vi "Main.vi"(11 "Module Admin":refnum<class "Delacor_lib_QMH_Module Admin.lvclass">) -> ()   [LabVIEW 2022 SP3, in "Dummy.lvlib"]
doc: "This template is based off of the Queued Message Handler design pattern and the Queued Message Handler project template that ships with LabVIEW.\n\nThe main difference is that the queue is private to this module and communication between modules is performed via Broadcast and Request events.\n\nRequest events are wrapped in public API methods and are handled in the Event Handling Loop (EHL) of this VI. Any module can register for Broadcast events sent by this module. The EHL generates messages based on user interface actions.\n\nThe Message Handling Loop (MHL) processes messages generated by the EHL, or by other messages. The messages are string values, so new messages can be added easily to the Message Cases case structure in the MHL. Each message cluster can also provide an optional value for Message Data, which is a variant that can be converted to whatever message-specific data is required.\n____\nHAMPEL SOFTWARE ENGINEERING v2.6.0 (2023-12-19 10:54)"
uses:
  Dummy.lvlib
  <vilib>/Delacor/Delacor QMH/Libraries/Module Admin_class/Delacor_lib_QMH_Module Admin.lvclass
  Libraries/hse-libraries/Source/hse-dqmh/Controls/Module Display Scenarios.ctl
  Module Data--cluster.ctl
  Stop Argument--cluster.ctl
  <vilib>/Delacor/Delacor QMH/Libraries/Message Queue_class/Delacor_lib_QMH_Message Queue.lvclass/Delacor_lib_QMH_Message Queue.ctl
  <vilib>/Delacor/Delacor QMH/Libraries/Module Admin_class/Delacor_lib_QMH_Module Admin.lvclass/Delacor_lib_QMH_Module Admin.ctl
  Configure Argument--cluster.ctl
  Prepare Argument--cluster.ctl
  Request UI Display Argument--cluster.ctl
  Request UI Display (Reply Payload)--cluster.ctl
  <vilib>/Utility/miscctls.llb/LVPointTypeDef.ctl
  <vilib>/Delacor/Delacor QMH/Libraries/Message Queue_class/Delacor_lib_QMH_Enqueue Message (Single).vi
  <vilib>/Delacor/Delacor QMH/Libraries/Module Admin_class/Delacor_lib_QMH_Get External Launch.vi
  <vilib>/Utility/error.llb/Error Cluster From Error Code.vi
  <vilib>/ErrorRing/Error Ring.xnode
  <vilib>/Delacor/Delacor QMH/Libraries/Message Queue_class/Delacor_lib_QMH_Message Queue.lvclass
  Libraries/hse-libraries/Source/hse-configuration/config-ini/config-ini.lvclass
  Libraries/hse-libraries/Source/hse-dqmh/hse-dqmh.lvlib
  ExampleClone/ExampleClone.lvlib
  Framework/UI Manager/UI Manager.lvlib
panel:
  out "CLI Arguments":string[](array[string])
  in  "Btn_DisableClose":bool
  in  "Btn_EnableClose":bool
  in  "Btn_HideRTM":bool
  in  "Btn_ShowRTM":bool
  in  "Message":string
  in  "Btn Send ExampleMessage":bool
  in  "Btn Show ExampleClone BD":bool
  in  "Module Display Scenarios":T1
  in  "Btn Stop ExampleClone":bool
  in  "Btn Show ExampleClone UI":bool
  out "ExampleClone ID":i32
  in  "Btn Run ExampleClone":bool
  out "error out":errorcluster
  # "UI Demo Functions"
  # "The \"Dummy\" serves as an example of a module with HSE functionality added so it can be used inside from\nand with all the features of the HSE UI Framework.\n\nThe module features a \"Configure\" request which is automatically called from the UI Framework during\nload time. The \"Configure\" case in the MHL will then load any configuration that is needed for this module.\n\nThe module features a \"Prepare\" request which is used for preparing the module's front panel before\nshowing it. The \"Prepare\" case of the MHL is called from the \"Request UI Display\" case (which, in turn, is\ncalled by the UI Manager when loading this module into its subpanel).\n\nFurthermore, this module showcases a few of the UI Framework's features.\n\nFinally, this module facilitates the starting, stopping and  operating of an example cloneable module."
  # "Controls for operating an example cloneable module"
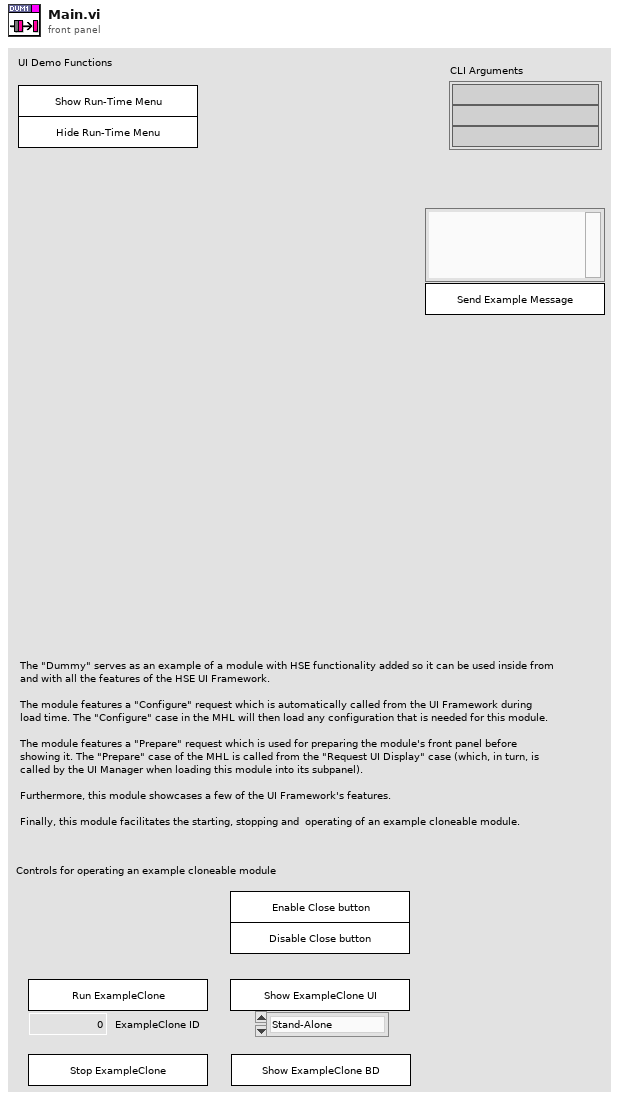
[diagram p1: front panel]
types:
  T1 = typedef "hse-dqmh.lvlib/Module Display Scenarios.ctl" = enum16{"Stand-Alone", "Managed"}
  T2 = typedef "Dummy.lvlib/Request Events--cluster.ctl" = cluster{"Stop Module":refnum<user-event>, "Show Panel":refnum<user-event>, "Hide Panel":refnum<user-event>, "Get Module Execution Status":refnum<user-event>, "Show Diagram":refnum<user-event>, "Configure":refnum<user-event>, "Prepare":refnum<user-event>, "Register for UI Login":refnum<user-event>, "Request UI Display":refnum<user-event>}
  T3 = typedef "UI Manager.lvlib/Broadcast Events--cluster.ctl" = cluster{"Module Did Init":refnum<user-event>, "Status Updated":refnum<user-event>, "Error Reported":refnum<user-event>, "Module Did Stop":refnum<user-event>, "Update Module Execution Status":refnum<user-event>, "System Message":refnum<user-event>, "Login":refnum<user-event>, "Key down":refnum<user-event>}
  T4 = typedef "Dummy.lvlib/Module Data--cluster.ctl" = cluster{"Status":string, "Clone ID's Ref":refnum<vi>}
  T5 = enum32{"invalid lock state", "Not Locked", "Locked (No Password)", "Password-protected"}
  T6 = typedef "Dummy.lvlib/Stop Argument--cluster.ctl" = cluster{"Origin":string, "Exit via Stop Module Req?":bool, "Wait for Module to stop?":bool}
  T7 = typedef "Dummy.lvlib/Configure Argument--cluster.ctl" = cluster{"Boolean":bool}
  T8 = typedef "Dummy.lvlib/Prepare Argument--cluster.ctl" = cluster{"Boolean":bool}
  T9 = typedef "Dummy.lvlib/Request UI Display Argument--cluster.ctl" = cluster{"Scenarios":T1, "Wait Notifier":refnum<notifier>, "wait for reply":bool}
  T10 = typedef "LVPointTypeDef.ctl" = cluster{"Horizontal":i16, "Vertical":i16}
  T11 = enum32{"Invalid", "Standard", "Closed", "Hidden", "Minimized", "Maximized"}
  T12 = typedef "Dummy.lvlib/Request UI Display (Reply Payload)--cluster.ctl" = cluster{"Accept?":bool, "Error":errorcluster}
  T13 = typedef "hse-dqmh.lvlib/System Message Source.ctl" = enum16{"module", "application", "network"}
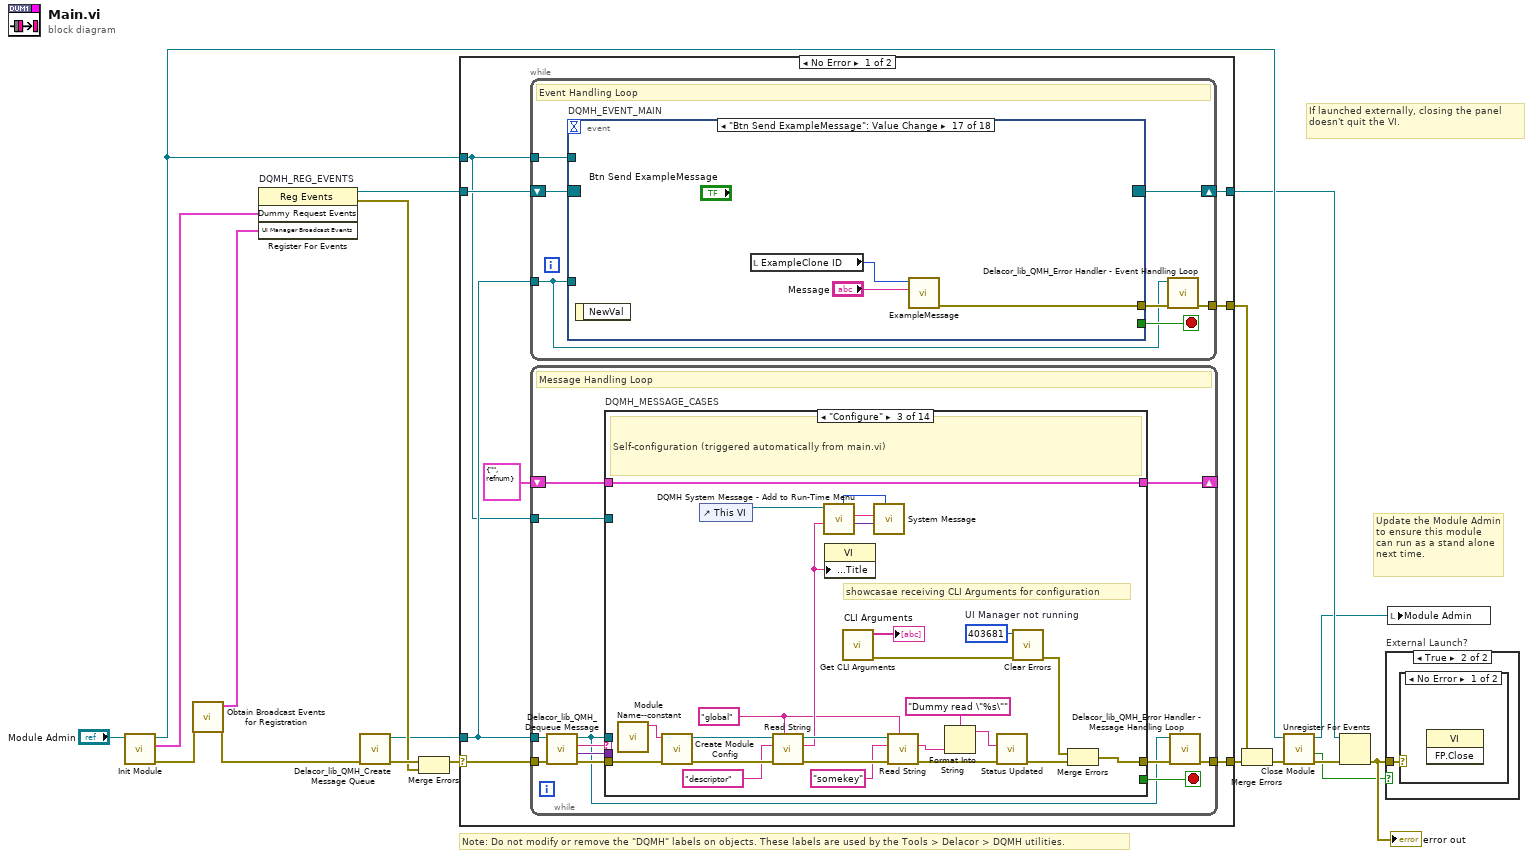
[diagram p0: block diagram]
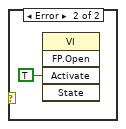
[diagram p3: hidden frame]
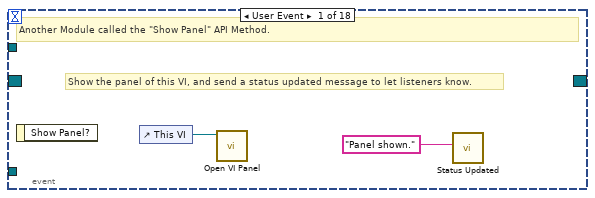
[diagram p4: hidden frame]
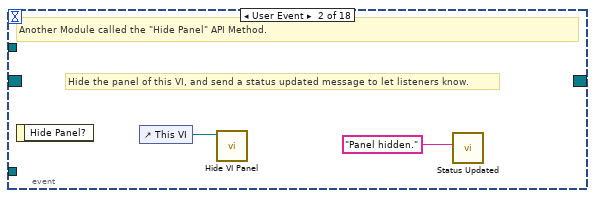
[diagram p5: hidden frame]
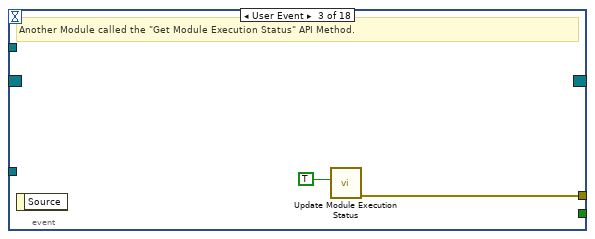
[diagram p6: hidden frame]
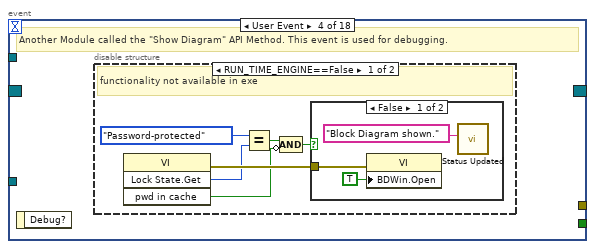
[diagram p7: hidden frame]
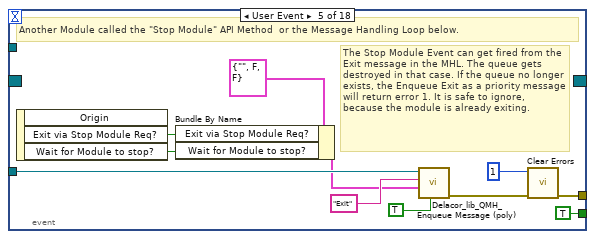
[diagram p10: hidden frame]
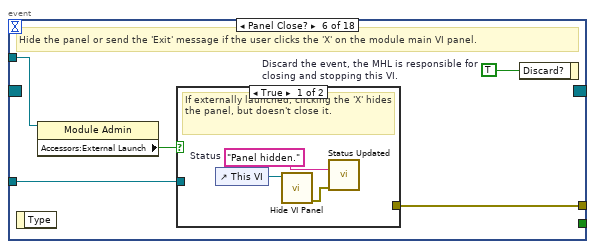
[diagram p11: hidden frame]
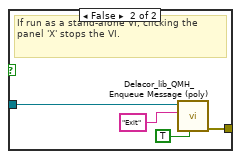
[diagram p12: hidden frame]
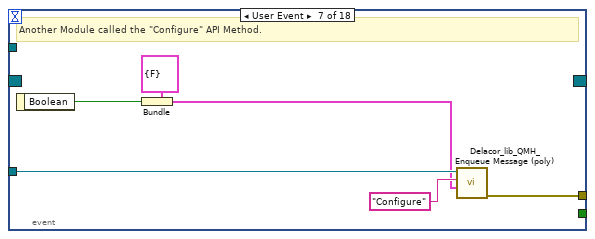
[diagram p13: hidden frame]
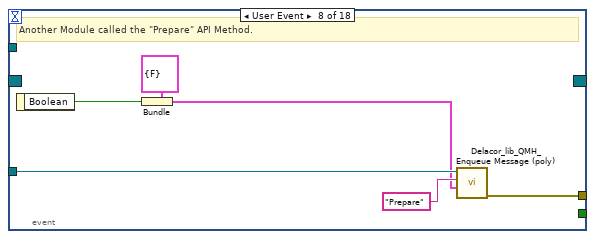
[diagram p14: hidden frame]
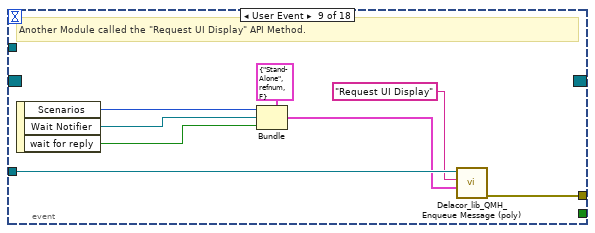
[diagram p15: hidden frame]
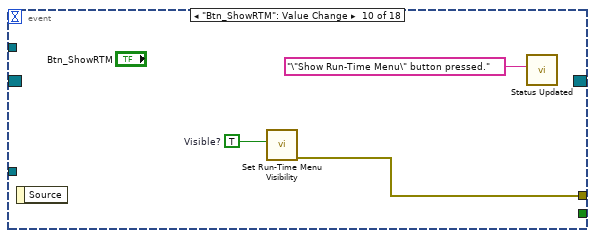
[diagram p16: hidden frame]
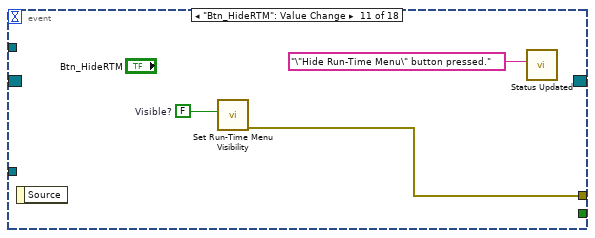
[diagram p17: hidden frame]
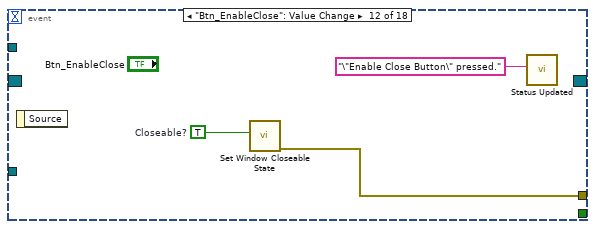
[diagram p18: hidden frame]
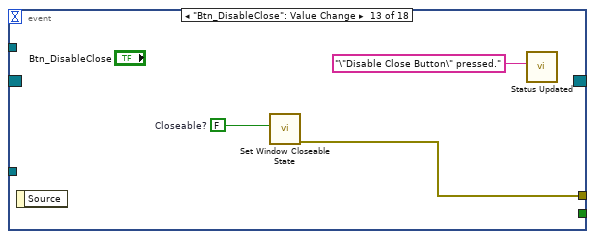
[diagram p19: hidden frame]
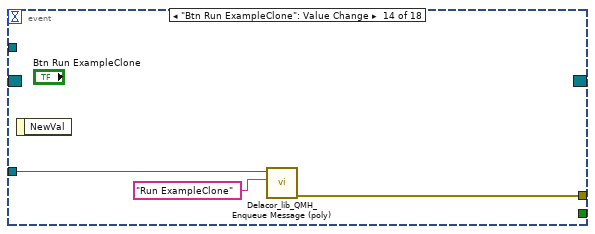
[diagram p20: hidden frame]
diagram:
  # "If launched externally, closing the panel doesn't quit the VI."
  # "Note: Do not modify or remove the \"DQMH\" labels on objects. These labels are used by the Tools > Delacor > DQMH utilities."
  # "Update the Module Admin to ensure this module can run as a stand alone next time."
  n1 = call "Init Module.vi"("Singleton Module Admin in"="Module Admin") -> ("error out"=w11:errorcluster, "Dummy Request Events"=w6:T2, "Singleton Module Admin out"=w9:refnum<class "Delacor_lib_QMH_Module Admin.lvclass">)  [unwired: 8 in]
  n2 = call "Obtain Broadcast Events for Registration.vi"("error in (no error)"=w11) -> ("error out"=w10:errorcluster, "UI Manager Broadcast Events"=w1:T3)  [unwired: 8 in, 1 out]
  n3 = register-events "DQMH_REG_EVENTS"(w6, w1) -> (reference out=w7:refnum<event-registration>, error out=w12:errorcluster)  [unwired: 2 in]
  n4 = call <vilib>:"Delacor_lib_QMH_Create Message Queue.vi"("error in"=w10) -> ("error out"=w14:errorcluster, "Message Queue"=w5:refnum<class "Delacor_lib_QMH_Message Queue.lvclass">)  [unwired: 9 in]
  n5 = Merge Errors(w14, w12) -> (w13:errorcluster)
  n6 = case shown="No Error" w13 {
    selector: w13 -> [w25 w297]
    tunnel: [w27 w297] -> w19
    tunnel: [w24 w294] -> w8
    tunnel: w7 -> [w22 w294]
    tunnel: w5 -> [w21 w289]
    tunnel: [w26 _] -> w17
    tunnel: w9 -> [w20 w290]
    frame No Error {
      n7 = while {
        tunnel: w21 -> [w28]
        shift-right: [w31] -> w24
        shift-left: w22 -> [w32]
        tunnel: [w33] -> w26
        tunnel: w20 -> [w29]
        stop <- w30 stop-if-true
        # "Event Handling Loop"
        n8 = event "DQMH_EVENT_MAIN" shown="[16] \"Btn Send ExampleMessage\": Value Change" {
          selector: w32 -> [_ _ _ _ _ _ _ _ _ _ _ _ _ _ _ _ _ _]
          dyn-events: [_ _ _ _ _ _ _ _ _ _ _ _ _ _ _ _ _ _] -> w31
          timeout: _ -> [_ _ _ _ _ _ _ _ _ _ _ _ _ _ _ _ _ _]
          tunnel: [_ _ _ _ TRUE ("Discard?") _ _ _ _ _ _ _ _ _ _ _ _ _] -> w30
          tunnel: w28 -> [_ _ _ _ w56 w63 w77 w83 w91 _ _ _ _ w105 w108 w112 _ w118]
          tunnel: [_ _ w40 _ w59 w65 w78 w84 w92 w95 w98 w101 w104 w107 w110 w114 w117 w120] -> w34
          tunnel: w29 -> [_ _ _ _ _ w62 _ _ _ _ _ _ _ _ _ _ _ _]
          event User Event {
            # "Show the panel of this VI, and send a status updated message to let listeners know."
            # "Another Module called the \"Show Panel\" API Method."
            n9 = event-data() -> ()  [unwired: 1 in, 1 out]
            n10 = control-ref of="This VI"() -> (w36:refnum<vi>)
            n11 = call "Open VI Panel.vi"("VI"=w36) -> ()  [unwired: 10 in, 1 out]
            n12 = call "Status Updated.vi"("Status"="Panel shown." ("format string")) -> ()  [unwired: 10 in, 1 out]
          }
          event User Event {
            # "Hide the panel of this VI, and send a status updated message to let listeners know."
            # "Another Module called the \"Hide Panel\" API Method."
            n13 = event-data() -> ()  [unwired: 1 in, 1 out]
            n14 = control-ref of="This VI"() -> (w38:refnum<vi>)
            n15 = call "Hide VI Panel.vi"("VI"=w38) -> ()  [unwired: 10 in, 1 out]
            n16 = call "Status Updated.vi"("Status"="Panel hidden." ("format string")) -> ()  [unwired: 10 in, 1 out]
          }
          event User Event {
            # "Another Module called the \"Get Module Execution Status\" API Method."
            n17 = event-data() -> ()  [unwired: 1 in, 1 out]
            n18 = call "Update Module Execution Status.vi"("Running?"=TRUE) -> ("error out"=w40:errorcluster)  [unwired: 10 in]
          }
          event User Event {
            # "Another Module called the \"Show Diagram\" API Method. This event is used for debugging."
            n19 = event-data() -> ()  [unwired: 1 in, 1 out]
            n20 = disable-structure shown="RUN_TIME_ENGINE==False" {
              frame condition #0 (active) {
                # "functionality not available in exe"
                n21 = invoke on="Invoke Node" class="VI" method="Lock State.Get"() -> (error out=w46:errorcluster, "Get Lock State"=w45:T5, "pwd in cache"=w42:bool)  [unwired: 4 in, 1 out]
                n22 = Equal?(x=T5."Password-protected", y=w45) -> (x = y?=w43:bool)
                n23 = Compound Arithmetic op=AND(w43, invert w42) -> (w41:bool)
                n24 = case shown="False" w41 {
                  tunnel: w46 -> [w49 _]
                  frame False {
                    n25 = property on="Property Node" class="VI"(error in=w49, "BDWin.Open"=TRUE ("Block Diagram Window:Open")) -> ()  [unwired: 1 in, 2 out]
                    n26 = call "Status Updated.vi"("Status"="Block Diagram shown." ("format string")) -> ()  [unwired: 10 in, 1 out]
                  }
                  frame True {
                    # "Password-protected VI, and the password is not in the cache. Do not show the diagram."
                  }
                }
              }
              frame condition #1 {
              }
            }
          }
          event User Event {
            # "The Stop Module Event can get fired from the Exit message in the MHL. The queue gets destroyed in that case. If the queue no longer exists, the Enqueue Exit as a priority message will return error 1. It is safe to ignore, because the module is already exiting."
            # "Another Module called the \"Stop Module\" API Method  or the Message Handling Loop below."
            n27 = event-data() -> ("Exit via Stop Module Req?"=w52:bool, "Wait for Module to stop?"=w51:bool)  [unwired: 1 in, 1 out]
            n28 = Bundle By Name(cluster=T6 {"Origin"="", "Exit via Stop Module Req?"=FALSE, "Wait for Module to stop?"=FALSE} ("Stop Argument"), "Exit via Stop Module Req?"=w52, "Wait for Module to stop?"=w51) -> (w50:T6)
            n29 = call-poly <vilib>:"Delacor_lib_QMH_Enqueue Message (poly).vi"("Priority Message? (F)"=TRUE, "Message Data"=w50, "Message"="Exit", "Message Queue in"=w56) -> ("error out"=w60:errorcluster)  [unwired: 6 in, 1 out]
            n30 = call <vilib>:"Clear Errors.vi"("error in (no error)"=w60, "specific error code to clear (0: all)"=1) -> ("error out"=w59:errorcluster)  [unwired: 4 in, 1 out]
          }
          event Panel Close? {
            w64 = TRUE  # Discard the event, the MHL is responsible for closing and stopping this VI.
            # "Hide the panel or send the 'Exit' message if the user clicks the 'X' on the module main VI panel."
            n31 = event-data() -> ()  [unwired: 1 in, 1 out]
            n32 = property on="Property Node" class="Module Admin"(reference=w62) -> ("Accessors:External Launch"=w61:bool)  [unwired: 1 in, 2 out]
            n33 = case shown="True" w61 {
              tunnel: w63 -> [_ w71]
              tunnel: [_ w72] -> w65
              frame True {
                w67 = "Panel hidden."  # Status
                # "If externally launched, clicking the 'X' hides the panel, but doesn't close it."
                n34 = control-ref of="This VI"() -> (w68:refnum<vi>)
                n35 = call "Hide VI Panel.vi"("VI"=w68) -> ("error out"=w66:errorcluster)  [unwired: 10 in]
                n36 = call "Status Updated.vi"("error in (no error)"=w66, "Status"=w67) -> ()  [unwired: 9 in, 1 out]
              }
              frame False {
                # "If run as a stand-alone VI, clicking the panel 'X' stops the VI."
                n37 = call-poly <vilib>:"Delacor_lib_QMH_Enqueue Message (poly).vi"("Priority Message? (F)"=TRUE, "Message"="Exit", "Message Queue in"=w71) -> ("error out"=w72:errorcluster)  [unwired: 7 in, 1 out]
              }
            }
            n38 = event-data ("Event Filter Node")("Discard?"=w64) -> ()  [unwired: 1 in, 1 out]
          }
          event User Event {
            # "Another Module called the \"Configure\" API Method."
            n39 = event-data() -> ("Boolean"=w73:bool)  [unwired: 1 in]
            n40 = Bundle(cluster=T7 {"Boolean"=FALSE} ("Configure Argument"), "Boolean"=w73) -> (w74:T7)
            n41 = call-poly <vilib>:"Delacor_lib_QMH_Enqueue Message (poly).vi"("Message Data"=w74, "Message"="Configure", "Message Queue in"=w77) -> ("error out"=w78:errorcluster)  [unwired: 7 in, 1 out]
          }
          event User Event {
            # "Another Module called the \"Prepare\" API Method."
            n42 = event-data() -> ("Boolean"=w79:bool)  [unwired: 1 in]
            n43 = Bundle(cluster=T8 {"Boolean"=FALSE} ("Prepare Argument"), "Boolean"=w79) -> (w80:T8)
            n44 = call-poly <vilib>:"Delacor_lib_QMH_Enqueue Message (poly).vi"("Message Data"=w80, "Message"="Prepare", "Message Queue in"=w83) -> ("error out"=w84:errorcluster)  [unwired: 7 in, 1 out]
          }
          event User Event {
            # "Another Module called the \"Request UI Display\" API Method."
            n45 = event-data() -> ("Scenarios"=w87:T1, "Wait Notifier"=w86:refnum<notifier>, "wait for reply"=w85:bool)  [unwired: 1 in]
            n46 = Bundle(cluster=T9 {"Scenarios"=enum."Stand-Alone", "Wait Notifier"=refnum, "wait for reply"=FALSE} ("Display Module UI Argument"), "Scenarios"=w87, "Wait Notifier"=w86, "wait for reply"=w85) -> (w88:T9)
            n47 = call-poly <vilib>:"Delacor_lib_QMH_Enqueue Message (poly).vi"("Message Data"=w88, "Message"="Request UI Display", "Message Queue in"=w91) -> ("error out"=w92:errorcluster)  [unwired: 7 in, 1 out]
          }
          event "Btn_ShowRTM": Value Change {
            w94 = TRUE  # Visible?
            n48 = event-data() -> ()  [unwired: 1 in, 1 out]
            n49 = call "Set Run-Time Menu Visibility.vi"("Visible?"=w94) -> ("error out"=w95:errorcluster)  [unwired: 10 in]
            n50 = call "Status Updated.vi"("Status"="\"Show Run-Time Menu\" button pressed.") -> ()  [unwired: 10 in, 1 out]
          }
          event "Btn_HideRTM": Value Change {
            w97 = FALSE  # Visible?
            n51 = event-data() -> ()  [unwired: 1 in, 1 out]
            n52 = call "Set Run-Time Menu Visibility.vi"("Visible?"=w97) -> ("error out"=w98:errorcluster)  [unwired: 10 in]
            n53 = call "Status Updated.vi"("Status"="\"Hide Run-Time Menu\" button pressed.") -> ()  [unwired: 10 in, 1 out]
          }
          event "Btn_EnableClose": Value Change {
            w100 = TRUE  # Closeable?
            n54 = event-data() -> ()  [unwired: 1 in, 1 out]
            n55 = call "Set Window Closeable State.vi"("Closeable?"=w100) -> ("error out"=w101:errorcluster)  [unwired: 10 in]
            n56 = call "Status Updated.vi"("Status"="\"Enable Close Button\" pressed.") -> ()  [unwired: 10 in, 1 out]
          }
          event "Btn_DisableClose": Value Change {
            w103 = FALSE  # Closeable?
            n57 = event-data() -> ()  [unwired: 1 in, 1 out]
            n58 = call "Set Window Closeable State.vi"("Closeable?"=w103) -> ("error out"=w104:errorcluster)  [unwired: 10 in]
            n59 = call "Status Updated.vi"("Status"="\"Disable Close Button\" pressed.") -> ()  [unwired: 10 in, 1 out]
          }
          event "Btn Run ExampleClone": Value Change {
            n60 = event-data() -> ()  [unwired: 1 in, 1 out]
            n61 = call-poly <vilib>:"Delacor_lib_QMH_Enqueue Message (poly).vi"("Message"="Run ExampleClone", "Message Queue in"=w105) -> ("error out"=w107:errorcluster)  [unwired: 8 in, 1 out]
          }
          event "Btn Show ExampleClone BD": Value Change {
            n62 = event-data() -> ()  [unwired: 1 in, 1 out]
            n63 = call-poly <vilib>:"Delacor_lib_QMH_Enqueue Message (poly).vi"("Message"="Show ExampleClone BD", "Message Queue in"=w108) -> ("error out"=w110:errorcluster)  [unwired: 8 in, 1 out]
          }
          event "Btn Show ExampleClone UI": Value Change {
            n64 = event-data() -> ()  [unwired: 1 in, 1 out]
            n65 = call-poly <vilib>:"Delacor_lib_QMH_Enqueue Message (poly).vi"("Message Data"="Module Display Scenarios", "Message"="Display ExampleClone UI", "Message Queue in"=w112) -> ("error out"=w114:errorcluster)  [unwired: 7 in, 1 out]
          }
          event "Btn Send ExampleMessage": Value Change {
            n66 = event-data() -> ()  [unwired: 1 in, 1 out]
            n67 = local read "ExampleClone ID"() -> (w115:i32)
            n68 = call "ExampleMessage.vi"("ExampleMessage"="Message", "Module ID"=w115) -> ("error out"=w117:errorcluster)  [unwired: 9 in]
          }
          event "Btn Stop ExampleClone": Value Change {
            n69 = event-data() -> ()  [unwired: 1 in, 1 out]
            n70 = call-poly <vilib>:"Delacor_lib_QMH_Enqueue Message (poly).vi"("Message"="Stop ExampleClone", "Message Queue in"=w118) -> ("error out"=w120:errorcluster)  [unwired: 8 in, 1 out]
          }
        }
        n71 = call-dynamic "Delacor_lib_QMH_Error Handler - Event Handling Loop.vi"("error in"=w34, "Message Queue in"=w28) -> ("dup error in"=w33:errorcluster)  [unwired: 8 in, 1 out]
      }
      n72 = while {
        tunnel: w21 -> [w123]
        shift-right: [w127] -> _
        shift-left: T4 {"Status"="", "Clone ID's Ref"=refnum} ("Data Cluster") -> [w128]
        tunnel: w25 -> [w131]
        tunnel: [w129] -> w27
        tunnel: w20 -> [w121]
        stop <- w126 stop-if-true
        # "Message Handling Loop"
        n73 = call-dynamic "Delacor_lib_QMH_Dequeue Message.vi"("error in"=w131, "Message Queue in"=w123) -> ("error out"=w130:errorcluster, "Message Data"=w124:variant, "Message"=w125:string, "Message Queue out"=w122:refnum<class "Delacor_lib_QMH_Message Queue.lvclass">)  [unwired: 6 in]
        n74 = case "DQMH_MESSAGE_CASES" shown="\"Configure\"" w125 {
          selector: w125 -> [_ _ _ _ _ _ _ _ _ _ _ _ _ w276]
          tunnel: w122 -> [_ _ _ _ _ _ _ _ _ _ _ w244 w267 _]
          tunnel: w130 -> [w149 w153 w159 w180 w191 w206 w214 w220 w229 w237 w241 w251 w274 w278]
          tunnel: [w148 w153 w163 w180 w189 w205 w216 w222 w231 w238 w241 w247 w271 w279] -> w132
          tunnel: w128 -> [w134 w152 w175 w179 w188 w204 w211 w219 w227 w235 w240 w246 w266 w277]
          tunnel: [w134 w152 w175 w179 w188 w204 w211 w219 w227 w235 w240 w246 w266 w277] -> w127
          tunnel: [_ _ _ _ _ _ _ _ _ _ _ _ w265 _] -> w126
          tunnel: w124 -> [_ _ _ _ w187 _ _ _ w226 _ _ w245 w264 _]
          tunnel: w121 -> [w139 _ _ _ _ _ _ _ _ _ _ w243 w259 _]
          frame "Initialize" {
            # "Initialize - Any operation that needs to be done before the module can receive messages. Synchronize Caller Events.vi will inform Start Module.vi that the module has launched and is ready to receive messages. Module Did Init.vi will broadcast that the module initialized."
            n75 = call "Synchronize Caller Events.vi"("error in (no error)"=w149, "Singleton Module Admin in"=w139) -> ("error out"=w147:errorcluster, "Singleton Module Admin out"=w136:refnum<class "Delacor_lib_QMH_Module Admin.lvclass">)  [unwired: 8 in]
            n76 = property on="Property Node" class="Module Admin"(reference=w136) -> ("Accessors:External Launch"=w143:bool)  [unwired: 1 in, 2 out]
            n77 = Select(t=T11."Hidden" ("State"), s=w143, f=T11."Standard" ("State")) -> (s? t:f=w140:T11)
            n78 = call "Module Name--constant.vi"() -> ("Module Name"=w146:string)  [unwired: 11 in]
            n79 = property on="Property Node" class="VI"("Front Panel.Title"=w146) -> (reference out=w145:refnum<vi>, error out=w151:errorcluster)  [unwired: 2 in]
            n80 = call "Module Name--constant.vi"() -> ("Module Name"=w137:string)  [unwired: 11 in]
            n81 = local write "ExampleClone ID"(-1 ("ExampleClone ID")) -> ()
            n82 = invoke on="Invoke Node" class="VI" method="FP.Open"(reference=w145, error in=w151, "State"=w140) -> (reference out=w144:refnum<vi>, error out=w150:errorcluster)  [unwired: 2 in, 3 out]
            n83 = call "Module Did Init.vi"("error in (no error)"=w147, "Initialized?"=TRUE, "Origin"=w137) -> ("error out"=w148:errorcluster)  [unwired: 8 in]
            n84 = invoke on="Invoke Node" class="VI" method="FP.Center"(reference=w144, error in=w150) -> ()  [unwired: 1 in, 3 out]
            n85 = property on="Pane" class="Pane"("Origin"=T10 {"Horizontal"=0, "Vertical"=0}) -> ()  [unwired: 2 in, 2 out]
          }
          frame "--- Module Specific ---" {
            # "Separator -- The following cases handle messages specific to this Module."
          }
          frame "Configure" {
            w160 = 403681  # UI Manager not running
            w155 = "global" ("Section")
            # "showcasae receiving CLI Arguments for configuration"
            # "Self-configuration (triggered automatically from main.vi)"
            n86 = call "Module Name--constant.vi"() -> ("Module Name"=w157:string)  [unwired: 11 in]
            n87 = call "Create Module Config.vi"("error in"=w159, "DQMH Module Name"=w157) -> ("error out"=w158:errorcluster, "config-ini out"=w156:refnum<class "config-ini.lvclass">)  [unwired: 8 in]
            n88 = control-ref of="This VI"() -> (w165:refnum<vi>)
            n89 = call-dynamic "Read String.vi"("Section"=w155, "error in"=w158, "Key"="descriptor", "config-base in"=w156) -> ("error out"=w176:errorcluster, "Value"=w166:string, "config-base out"=w167:refnum<class "config-ini.lvclass">)  [unwired: 5 in]
            n90 = call "DQMH System Message - Add to Run-Time Menu.vi"("Module Descriptor"=w166, "Main VI Reference"=w165) -> ("Payload"=w169:variant, "Identifier"=w168:string, "Source"=w170:T13)  [unwired: 7 in]
            n91 = property on="Property Node" class="VI"("Front Panel.Title"=w166) -> ()  [unwired: 2 in, 2 out]
            n92 = call "Get CLI Arguments.vi"() -> ("error out"=w162:errorcluster, "CLI Arguments"=→"CLI Arguments":string[])  [unwired: 9 in, 1 out]
            n93 = call "System Message.vi"("S. Message Source"=w170, "Payload"=w169, "Identifier"=w168) -> ()  [unwired: 8 in, 1 out]
            n94 = call-dynamic "Read String.vi"("Section"=w155, "error in"=w176, "Key"="somekey", "config-base in"=w167) -> ("error out"=w178:errorcluster, "Value"=w171:string)  [unwired: 5 in, 1 out]
            n95 = Format Into String(format string="Dummy read \"%s\"", w171) -> (resulting string=w172:string)  [unwired: 2 in, 1 out]
            n96 = call "Status Updated.vi"("error in (no error)"=w178, "Status"=w172) -> ("error out"=w177:errorcluster)  [unwired: 9 in]
            n97 = call <vilib>:"Clear Errors.vi"("error in (no error)"=w162, "specific error code to clear (0: all)"=w160) -> ("error out"=w161:errorcluster)  [unwired: 4 in, 1 out]
            n98 = Merge Errors(w161, w177) -> (w163:errorcluster)
          }
          frame "Prepare" {
            # "Prepare (the UI of the) module for display"
          }
          frame "Request UI Display" {
            # "Requests the module to display its UI as specified in <b>Scenario</b>:\n\"managed\" => in the UI Manager's subpanel\n\"stand-alone\" => as a separate window"
            n99 = Variant To Data(error in=w191, type=T9 {"Scenarios"=enum."Stand-Alone", "Wait Notifier"=refnum, "wait for reply"=FALSE} ("Request UI Display Argument"), Variant=w187) -> (data=w185:T9, error out=w190:errorcluster)
            n100 = Unbundle By Name(w185) -> ("Scenarios"=w181:T1, "Wait Notifier"=w184:refnum<notifier>, "wait for reply"=w183:bool)
            n101 = control-ref of="This VI"() -> (w182:refnum<vi>)
            n102 = case shown="\"Managed\"" w181 {
              tunnel: w182 -> [w193 w195]
              tunnel: [w194 w199] -> w192
              frame "Stand-Alone", Default {
                n103 = call "Open VI Panel.vi"("VI"=w193) -> ("error out"=w194:errorcluster)  [unwired: 10 in]
              }
              frame "Managed" {
                n104 = call "DQMH System Message - Ready for Display.vi"("Main VI Reference"=w195) -> ("Payload"=w198:variant, "Identifier"=w197:string, "Source"=w196:T13)  [unwired: 8 in]
                n105 = call "System Message.vi"("S. Message Source"=w196, "Payload"=w198, "Identifier"=w197) -> ("error out"=w199:errorcluster)  [unwired: 8 in]
              }
            }
            n106 = case shown="True" w183 {
              tunnel: w184 -> [_ w202]
              tunnel: w192 -> [_ w203]
              frame False {
              }
              frame True {
                n107 = Bundle By Name(cluster=T12 {"Accept?"=FALSE, "Error"={"status"=FALSE, "code"=0, "source"=""}} ("Request UI Display (Reply Payload)"), "Error"=w203) -> (w200:T12)
                n108 = Send Notification(notification=w200, notifier=w202) -> ()  [unwired: 1 in, 2 out]
              }
            }
            n109 = Merge Errors(w190, w192) -> (w189:errorcluster)
          }
          frame "---ExampleClone Functions---" {
            # "ExampleClone is a showcase for how the HSE DQMH functions work with cloneable modules"
            n110 = Merge Errors(w206) -> (w205:errorcluster)
          }
          frame "Run ExampleClone" {
            # "3. configure"
            # "2. register with framework"
            # "1. start module"
            # "ExampleClone is a showcase for how the HSE DQMH functions work with cloneable modules.\nBeware: It's important to register the clone with the Framework!"
            n111 = call "Start Module.vi"("error in (no error)"=w214) -> ("error out"=w215:errorcluster, "Wait for Event Sync?"=w210:bool, "Module ID"=w209:i32)  [unwired: 7 in, 1 out]
            n112 = call "Synchronize Module Events.vi"("error in (no error)"=w215, "Wait for Event Sync?"=w210, "Module ID"=w209) -> ("error out"=w217:errorcluster, "Module ID (dup)"=w208:i32)  [unwired: 7 in]
            "ExampleClone ID" <- w208
            n113 = control-ref of="This Application"() -> (w207:refnum<vi>)
            n114 = call "Register Clone with Framework.vi"("error in (no error)"=w217, "Application in"=w207) -> ("error out"=w213:errorcluster)  [unwired: 9 in]
            n115 = call "Configure.vi"("error in (no error)"=w213, "Module ID"=w208) -> ("error out"=w212:errorcluster)  [unwired: 9 in]
            n116 = Merge Errors(w212) -> (w216:errorcluster)
          }
          frame "Show ExampleClone BD" {
            # "ExampleClone is a showcase for how the HSE DQMH functions work with cloneable modules"
            n117 = local read "ExampleClone ID"() -> (w218:i32)
            n118 = call "Show Diagram.vi"("error in (no error)"=w220, "Module ID"=w218) -> ("error out"=w221:errorcluster)  [unwired: 9 in]
            n119 = Merge Errors(w221) -> (w222:errorcluster)
          }
          frame "Display ExampleClone UI" {
            # "ExampleClone is a showcase for how the HSE DQMH functions work with cloneable modules"
            n120 = local read "ExampleClone ID"() -> (w223:i32)
            n121 = Variant To Data(error in=w229, type=Module_Display_Scenarios."Stand-Alone" ("Module Display Scenarios"), Variant=w226) -> (data=w224:T1, error out=w228:errorcluster)
            n122 = call "Request UI Display.vi"("error in (no error)"=w228, "Scenario"=w224, "Module ID"=w223) -> ("error out"=w230:errorcluster)  [unwired: 7 in, 1 out]
            n123 = Merge Errors(w230) -> (w231:errorcluster)
          }
          frame "Stop ExampleClone" {
            w232 = TRUE  # Wait for Module to stop? (F)
            # "ExampleClone is a showcase for how the HSE DQMH functions work with cloneable modules"
            n124 = local read "ExampleClone ID"() -> (w234:i32)
            n125 = call "Module Name--constant.vi"() -> ("Module Name"=w233:string)  [unwired: 11 in]
            n126 = call "Stop Module.vi"("error in (no error)"=w237, "Wait for Module to stop? (F)"=w232, "Origin"=w233, "Module ID"=w234) -> ("error out"=w236:errorcluster)  [unwired: 7 in]
            n127 = flat-sequence {
              tunnel: w236 -> [_]
              frame #0 {
                n128 = local write "ExampleClone ID"(-1 ("ExampleClone ID")) -> ()
              }
            }
            n129 = Merge Errors(w236) -> (w238:errorcluster)
          }
          frame "--- Exit and Error Handling---" {
            # "Separator - The following cases handle errors and exit messages."
          }
          frame "Error" {
            # "#CodeRecommended - If you ever change the name of this \"Error\" message, you'll need to update the name in the Check Loop Error.vi as well."
            # "#CodeRecommended - If the module is running in standalone mode (External Launch = FALSE), this code will pop up an error dialog and call the 'Exit' message if an error occurs. Add more fine-grained error handling here."
            # "Error - Check the error message data and respond accordingly. This message is sent by the \"Error Handler\" VIs at the end of each loop in this application."
            n130 = property on="Property Node" class="Module Admin"(reference=w243) -> ("Accessors:External Launch"=w242:bool)  [unwired: 1 in, 2 out]
            n131 = Variant To Data(error in=w251, type=errorcluster {"status"=FALSE, "code"=0, "source"=""} ("error constant"), Variant=w245) -> (data=w252:errorcluster, error out=w249:errorcluster)
            n132 = call "Error Reported.vi"("Error"=w252) -> ()  [unwired: 10 in, 1 out]
            n133 = case shown="False" w242 {
              tunnel: [w256 _] -> w248
              tunnel: w244 -> [w255 _]
              tunnel: w252 -> [_ _]
              frame False {
                # "If the module is running standalone, then pop up an error dialog and call the \"Exit\" message."
                n134 = call-poly <vilib>:"Delacor_lib_QMH_Enqueue Message (poly).vi"("Priority Message? (F)"=TRUE, "Message"="Exit", "Message Queue in"=w255) -> ("error out"=w256:errorcluster)  [unwired: 7 in, 1 out]
              }
              frame True {
                # "If the module was launched externally, calling the Error Reported broadcast VI is the only action performed by the \"Error\" message. The module's caller can then process the error appropriately."
              }
            }
            n135 = Merge Errors(w249, w248) -> (w247:errorcluster)
            n136 = local write "error out"(w247) -> ()
          }
          frame "Exit" {
            w257 = -1  # Module ID
            w263 = 91  # 91: not all Exit messages will have an argument
            w265 = TRUE  # Stop the VI
            # "Release the message queue reference"
            # "Exit - Exit the application."
            n137 = Variant To Data(error in=w274, type=T6 {"Origin"="", "Exit via Stop Module Req?"=FALSE, "Wait for Module to stop?"=FALSE} ("Stop Argument"), Variant=w264) -> (data=w261:T6, error out=w270:errorcluster)
            n138 = call <vilib>:"Clear Errors.vi"("error in (no error)"=w270, "specific error code to clear (0: all)"=w263) -> ("error out"=w273:errorcluster)  [unwired: 4 in, 1 out]
            n139 = control-ref of="This VI"() -> (w260:refnum<vi>)
            n140 = call "Module Name--constant.vi"() -> ("Module Name"=w258:string)  [unwired: 11 in]
            n141 = call "Stop Module.vi"("Origin"=w258, "Module ID"=w257) -> ("error out"=w268:errorcluster)  [unwired: 9 in]
            n142 = call-dynamic "Delacor_lib_QMH_Release Message Queue.vi"("error in"=w273, "Message Queue"=w267) -> ("error out"=w272:errorcluster)  [unwired: 9 in]
            n143 = call "Handle Exit.vi"("Stop Argument"=w261, "Admin in"=w259, "VI reference"=w260) -> ("error out"=w269:errorcluster)  [unwired: 7 in, 1 out]
            n144 = Merge Errors(w272, w269, w268) -> (w271:errorcluster)
            n145 = call "Error Reported.vi"("Error"=w271) -> ()  [unwired: 10 in, 1 out]
          }
          frame Default {
            # "'Default' case only runs if there is a message that isn't defined in any of the other cases.  Output a programming error."
            n146 = call "Module Name--constant.vi"() -> ("Module Name"=w275:string)  [unwired: 11 in]
            n147 = xnode "Error Ring"("parameter 0"=w276, "parameter 1"=w275) -> ("error out"=w280:errorcluster)
            n148 = Merge Errors(w278, w280) -> (w279:errorcluster)
          }
        }
        n149 = call-dynamic "Delacor_lib_QMH_Error Handler - Message Handling Loop.vi"("error in"=w132, "Message Queue in"=w122) -> ("dup error in"=w129:errorcluster)  [unwired: 8 in, 1 out]
      }
    }
    frame Error {
      # "Synchronize Caller Events.vi will inform Start Module.vi that the module has launched and will let the code calling Start Module.vi register for broadcasts and would permit the caller receive the broadcast that an error occurred at launch time."
      n150 = call "Synchronize Caller Events.vi"("Singleton Module Admin in"=w290) -> ("error out"=w295:errorcluster)  [unwired: 9 in, 1 out]
      n151 = call-dynamic "Delacor_lib_QMH_Release Message Queue.vi"("Message Queue"=w289) -> ()  [unwired: 10 in, 1 out]
      n152 = call "Module Name--constant.vi"() -> ("Module Name"=w293:string)  [unwired: 11 in]
      n153 = Format Into String(format string="An error occurred during initialization. %s is no longer running.", w293) -> (resulting string=w291:string)  [unwired: 2 in, 1 out]
      n154 = Merge Errors(w297, w295) -> (w296:errorcluster)
      n155 = call "Error Reported.vi"("Additional Information"=w291, "Error"=w296) -> ()  [unwired: 9 in, 1 out]
    }
  }
  n156 = Merge Errors(w17, w19) -> (w16:errorcluster)
  n157 = call "Close Module.vi"("error in (no error)"=w16, "Module Admin in"=w9) -> ("error out"=w18:errorcluster, "External Launch"=w2:bool, "Module Admin out"=w3:refnum<class "Delacor_lib_QMH_Module Admin.lvclass">)  [unwired: 7 in]
  n158 = Unregister For Events(event registration refnum=w8, error in=w18) -> (error out=w15:errorcluster)
  "error out" <- w15
  n159 = case "External Launch?" shown="True" w2 {
    tunnel: w15 -> [_ w298]
    frame False {
    }
    frame True {
      n160 = case shown="No Error" w298 {
        frame No Error {
          n161 = invoke on="Invoke Node" class="VI" method="FP.Close"() -> ()  [unwired: 3 in, 3 out]
        }
        frame Error {
          n162 = invoke on="Invoke Node" class="VI" method="FP.Open"("Activate"=TRUE ("Activate?")) -> ()  [unwired: 4 in, 5 out]
        }
      }
    }
  }
  n163 = local write "Module Admin"(w3) -> ()
